vi "queue_state_&_argument.vi"(6 "Priority":bool, 8 "error in (no error)":errorcluster, 10 "list state:argument":string, 11 "Queue in":refnum<queue>) -> (0 "error out":errorcluster, 3 "Queue out":refnum<queue>)   [LabVIEW 2015]
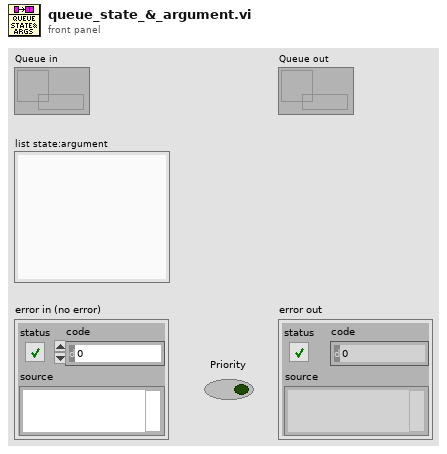
[diagram p1: front panel]
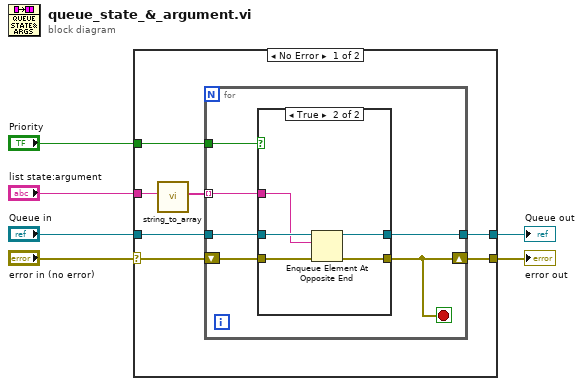
[diagram p0: block diagram]
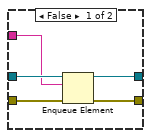
[diagram p2: hidden frame]
diagram:
  n1 = case shown="No Error" "error in (no error)" {
    selector: "error in (no error)" -> [w12 w31]
    tunnel: [w11 w31] -> w3
    tunnel: "list state:argument" -> [w13 _]
    tunnel: "Queue in" -> [w10 w30]
    tunnel: [w9 w30] -> w6
    tunnel: "Priority" -> [w7 _]
    frame No Error {
      n2 = call "string_to_array.vi"("list state:arg"=w13) -> ("state:arg array"=w8:string[])  [unwired: 10 in]
      n3 = for {
        shift-right: [w15] -> w11
        shift-left: w12 -> [w19]
        tunnel: w10 -> [w18]
        tunnel: [w17] -> w9
        tunnel: w8 -> [w16] mode=indexing
        tunnel: w7 -> [w14]
        stop <- w15 stop-if-true
        n4 = case shown="True" w14 {
          tunnel: w19 -> [w24 w29]
          tunnel: w18 -> [w23 w27]
          tunnel: [w22 w26] -> w17
          tunnel: w16 -> [w21 w25]
          tunnel: [w20 w28] -> w15
          frame False {
            n5 = Enqueue Element(queue=w23, element=w21, error in (no error)=w24) -> (queue out=w22:refnum<queue>, error out=w20:errorcluster)  [unwired: 1 in, 1 out]
          }
          frame True {
            n6 = Enqueue Element At Opposite End(queue=w27, element=w25, error in (no error)=w29) -> (queue out=w26:refnum<queue>, error out=w28:errorcluster)  [unwired: 1 in, 1 out]
          }
        }
      }
    }
    frame Error {
    }
  }
  "error out" <- w3
  "Queue out" <- w6
